vi "SubSystems.vi"(8 "error in":errorcluster) -> ()   [LabVIEW 2015]
doc: "This VI calls the various robot subsystems that will then run in parallel. New subSystems will automatlically script code to make the call."
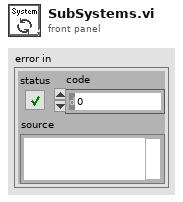
[diagram p1: front panel]
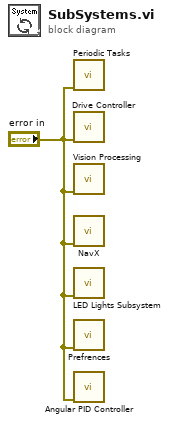
[diagram p0: block diagram]
diagram:
  n1 = call "Periodic Tasks.vi"("error in"="error in") -> ()  [unwired: 1 in, 10 out]
  n2 = call "Drive Controller.vi"("error in"="error in") -> ()  [unwired: 11 in]
  n3 = call "Vision Processing.vi"("error in (no error)"="error in") -> ()  [unwired: 7 in]
  n4 = call "NavX.vi"("error in"="error in") -> ()  [unwired: 11 in]
  n5 = call "LED Lights Subsystem.vi"("error in"="error in") -> ()  [unwired: 11 in]
  n6 = call "Prefrences.vi"("error in"="error in") -> ()  [unwired: 11 in]
  n7 = call "Angular PID Controller.vi"("error in"="error in") -> ()  [unwired: 11 in]
